vi "Write to end emibin file FUNKER INTE.vi"(0 "refnum in":refnum<file>, 7 "Data":variant, 11 "error in (no error)":errorcluster) -> (4 "refnum out":refnum<file>, 15 "error out":errorcluster)   [LabVIEW 2011]
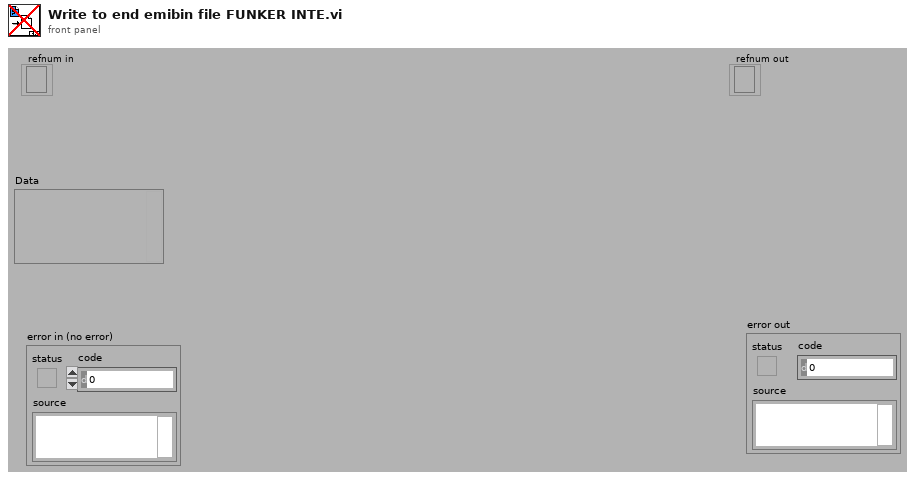
[diagram p1: front panel]
types:
  T1 = enum16{"big-endian, network order", "native, host order", "little-endian"}
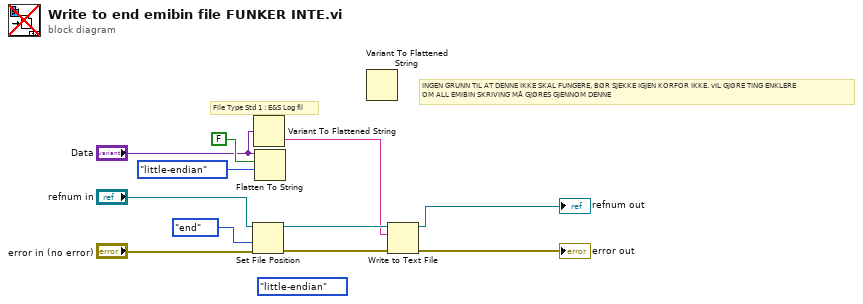
[diagram p0: block diagram]
diagram:
  (unwired) T1."little-endian" ("byte order (0:big-endian, network order)")
  # "INGEN GRUNN TIL AT DENNE IKKE SKAL FUNGERE, BØR SJEKKE IGJEN KORFOR IKKE. vIL GJØRE TING ENKLERE\nOM ALL EMIBIN SKRIVING MÅ GJØRES GJENNOM DENNE"
  # "File Type Std 1 : E&S Log fil"
  n1 = Set File Position(refnum="refnum in", from (0:start)=enum16{"start", "end", "current"}."end", error in="error in (no error)") -> (refnum out=w3:refnum<file>, error out=w8:errorcluster)  [unwired: 1 in]
  n2 = Variant To Flattened String(Variant="Data") -> (data string=w1:string)  [unwired: 1 out]
  n3 = Flatten To String(anything="Data", prepend array or string size? (T)=FALSE, byte order (0:big-endian, network order)=T1."little-endian") -> ()  [unwired: 1 in, 3 out]
  n4 = Variant To Flattened String() -> ()  [unwired: 1 in, 2 out]
  n5 = Write to Text File(file (use dialog)=w3, text=w1, error in=w8) -> (refnum out=→"refnum out":refnum<file>, error out=→"error out":errorcluster)  [unwired: 1 in, 1 out]
